vi "Untitled 1.vi"() -> ()   [LabVIEW 2016]
panel:
  in  "x":dbl(knob) scale=-100.0..100.0
  out "max(x,y)":dbl
  in  "reset 2":bool
  in  "reset":bool
  out "count":i32
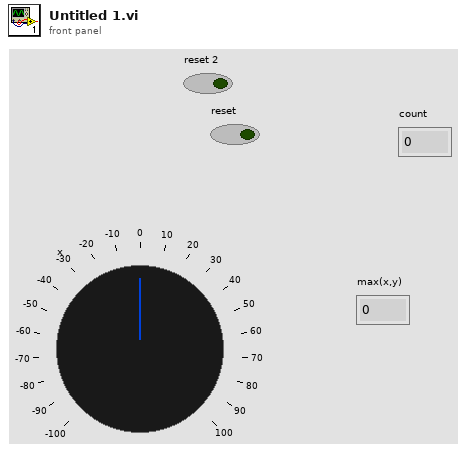
[diagram p1: front panel]
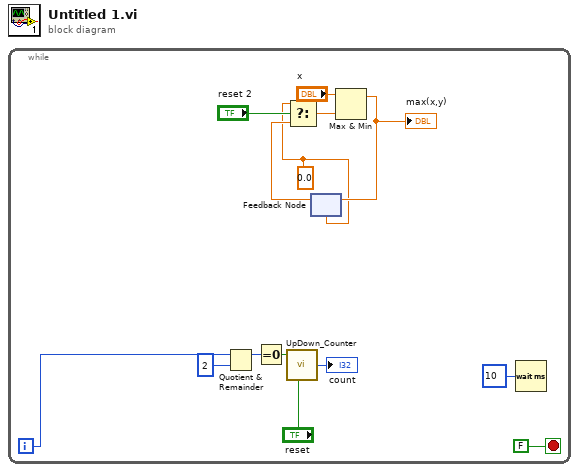
[diagram p0: block diagram]
diagram:
  n1 = while {
    i -> [w10]
    stop <- FALSE stop-if-true
    w2 = 0.0
    n2 = Quotient & Remainder(x=w10, y=2) -> (x-y*floor(x/y)=w8:i32)  [unwired: 1 out]
    n3 = Equal To 0?(x=w8) -> (x = 0?=w7:bool)
    n4 = call <userlib>:"UpDown_Counter.vi"("up"=w7, "reset"="reset") -> ("count"=→"count":i32)  [unwired: 3 in]
    n5 = feedback #1(w2) -> (w4:dbl)
    n6 = Select(t=w2, s="reset 2", f=w4) -> (s? t:f=w3:dbl)
    n7 = Max & Min(x="x", y=w3) -> (max(x,y)=w6:dbl)  [unwired: 1 out]
    "max(x,y)" <- w6
    n8 = feedback-in #1(w6) -> ()
    n9 = Wait (ms)(milliseconds to wait=u32 10) -> ()  [unwired: 1 out]
  }
